vi "Configure Smoothing.vi"(5 "Mode (0: Smooth Points)":i32(ring) items=["Smooth Points", "Smooth Aperture"], 6 "Smooth Aperture (1.5 %)":dbl=1.5, 7 "Smooth Points (3)":dbl=3.0, 8 "error in (no error)":errorcluster, 9 "Enable Smooth (F: Disable)":bool, 10 "Channel (1)":i32=1, 11 "VISA resource name":refnum<visa-resource-name>) -> (0 "error out":errorcluster, 3 "VISA resource name out":refnum<visa-resource-name>)   [LabVIEW 2018, in "Keysight PNA Series.lvlib"]
doc: "Configures point-to-point smoothing."
uses:
  Keysight PNA Series.lvlib
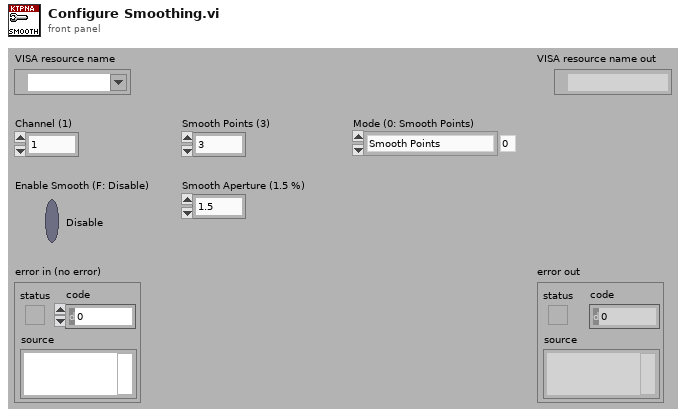
[diagram p1: front panel]
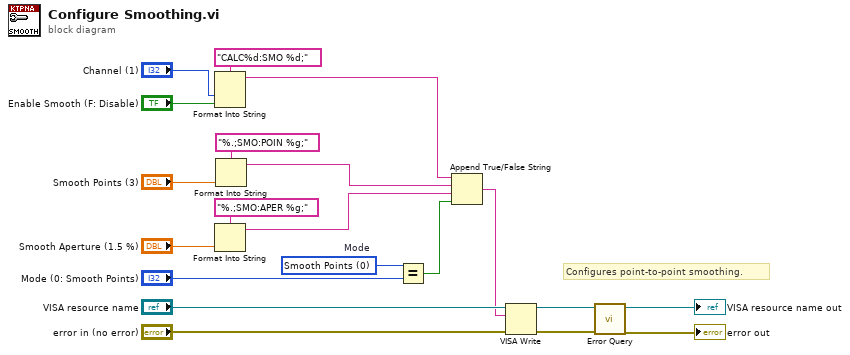
[diagram p0: block diagram]
diagram:
  w4 = 0 items=["Smooth Points", "Smooth Aperture"]  # Mode
  # "Configures point-to-point smoothing."
  n1 = Format Into String(format string="CALC%d:SMO %d;", "Channel (1)", "Enable Smooth (F: Disable)") -> (resulting string=w7:string)  [unwired: 2 in, 1 out]
  n2 = Format Into String(format string="%.;SMO:APER %g;", "Smooth Aperture (1.5 %)") -> (resulting string=w5:string)  [unwired: 2 in, 1 out]
  n3 = Format Into String(format string="%.;SMO:POIN %g;", "Smooth Points (3)") -> (resulting string=w6:string)  [unwired: 2 in, 1 out]
  n4 = Equal?(x=w4, y="Mode (0: Smooth Points)") -> (x = y?=w2:bool)
  n5 = Append True/False String(1:w2, 2:w5, 3:w6, 4:w7) -> (0:w1:string)
  n6 = VISA Write(VISA resource name="VISA resource name", write buffer=w1, error in (no error)="error in (no error)") -> (VISA resource name out=w12:refnum<visa-resource-name>, error out=w11:errorcluster)  [unwired: 1 out]
  n7 = call "Error Query.vi"("error in (no error)"=w11, "VISA resource name"=w12) -> ("error out"=→"error out":errorcluster, "VISA resource name out"=→"VISA resource name out":refnum<visa-resource-name>)  [unwired: 6 in, 2 out]
